vi "endianSwitch.vi"(11 "U16 array in":u16[](array[numeric])) -> (3 "U16 array out":u16[](array[numeric]))   [LabVIEW 2020]
doc: "Exchange odd-indexed and even-indexed elements in <B>U16 array in</B>."
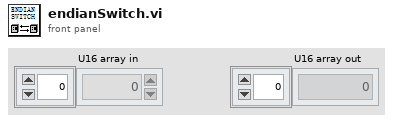
[diagram p1: front panel]
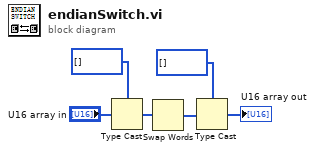
[diagram p0: block diagram]
diagram:
  n1 = Type Cast(type=u32[] [], x="U16 array in") -> (*(type *) &x=w4:u32[])
  n2 = Swap Words(1:w4) -> (0:w3:u32[])
  n3 = Type Cast(type=u16[] [], x=w3) -> (*(type *) &x=→"U16 array out":u16[])
